vi "Add Item to ListView by Text.vi"(8 "error in (no error)":errorcluster caption="错误输入（无错误）", 10 "Text":string, 11 "ListViewClass 输入":refnum<class "ListViewClass.lvclass"> caption="DNL_LabVIEW Object in") -> (0 "error out":errorcluster caption="错误输出", 3 "ListViewClass 输出":refnum<class "ListViewClass.lvclass"> caption="DNL_LabVIEW Object out")   [LabVIEW 2012, in "ListViewClass.lvclass"]
uses:
  ListViewClass.lvclass
  ListViewClass.lvclass/ListViewClass.ctl
  System.Windows.Forms
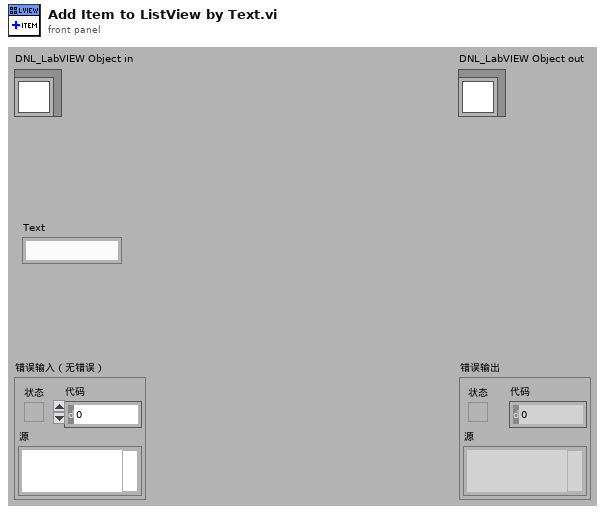
[diagram p1: front panel]
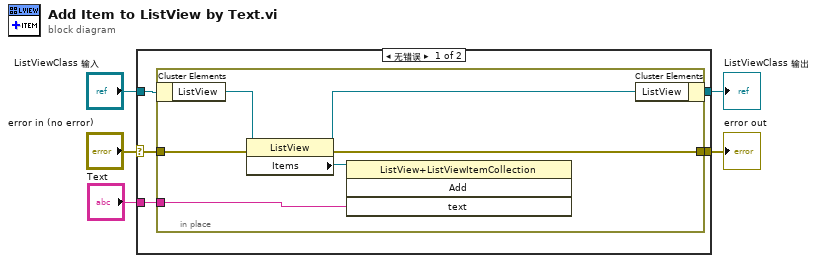
[diagram p0: block diagram]
diagram:
  n1 = case shown="无错误" "error in (no error)" {
    selector: "error in (no error)" -> [w7 w18]
    tunnel: [w6 w18] -> w4
    tunnel: [w8 w17] -> w2
    tunnel: "ListViewClass 输入" -> [w10 w17]
    tunnel: "Text" -> [w9 _]
    frame No Error {
      n2 = in-place {
        in-place-border: w9 -> [w13]
        in-place-border: w7 -> [w12]
        in-place-border: [w11] -> w6
        n3 = in-place-cluster #1(w10) -> ("ListView"=w16:refnum<k24>)
        n4 = property class="ListView"(reference=w16, error in=w12) -> (reference out=w15:refnum<k24>, error out=w11:errorcluster, "Items"=w14:refnum<k24>)
        n5 = invoke class="ListView+ListViewItemCollection" method="Add"(reference=w14, "text"=w13) -> ()  [unwired: 2 in, 4 out]
        n6 = in-place-cluster #1("ListView"=w15) -> (w8:refnum<class "ListViewClass.lvclass">)
      }
    }
    frame Error {
    }
  }
  "error out" <- w4
  "ListViewClass 输出" <- w2
